vi "FCE_TS_Action_InitControls.vi"(8 "err in":errorcluster) -> (0 "err out":errorcluster)   [LabVIEW 2017]
uses:
  FCE_TS_General_Libs/WL_Libs_V14.25/WL_Alarm_V14.00.llb/WL_Alarm_TypeDefClusterStatus.ctl
  FCE_TS_GUI_V001.llb/FCE_TS_GUI_TDefEnumMessages.ctl
  FCE_TS_Auto_V001.llb/FCE_TS_Auto_TDefCluster_AutomaticSetpoints.ctl
  FCE_TS_Globals_V001.llb/Globals_Settings_FCE_TS.vi
  FCE_TS_Globals_V001.llb/FCE_TS_Globals_Status.vi
  FCE_TS_Globals_V001.llb/FCE_TS_Globals_Referenzen.vi
  FCE_TS_Alarm_V001.llb/FCE_TS_Alarm_Globals.vi
  FCE_TS_Auto_V001.llb/FCE_TS_Auto_Globals.vi
  FCE_TS_General_Libs/WL_Libs_V14.25/WL_Alarm_V14.00.llb/WL_Alarm_Globals.vi
  FCE_TS_Datalog_V002.llb/FCE_TS_Datalog_Globals.vi
  FCE_TS_General_Libs/WL_Libs_V14.25/WL_Profile_V14.00.llb/WL_Profile_Globals.vi
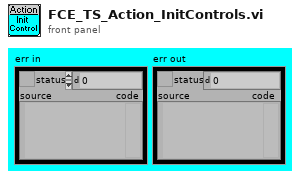
[diagram p1: front panel]
types:
  T1 = typedef "FCE_TS_Action_TDefEnumControl.ctl" = enum16{"Service", "Auto"}
  T2 = enum32{"Debug", "P&ID", "I/Os", "Regulator", "Datalog", "Automatic", "Charts", "CVM"}
  T3 = typedef "FCE_TS_GUI_TDefEnumMessages.ctl" = enum16{"Clear", "Add"}
  T4 = cluster{"Comment":string, "SamplingRate":u32, "Logging":bool, "FileName":string}
  T5 = typedef "FCE_TS_Auto_TDefCluster_AutomaticSetpoints.ctl" = cluster{"DC_Power":sgl, "AC_Power":sgl, "AC_Exists":bool, "Minute_Reserve":bool, "C_U_E_Soll":sgl, "Referenzpunkt_On":bool}
  T6 = typedef "WL_Alarm_TypeDefClusterStatus.ctl" = cluster{"NOTAUS":bool, "ABSCHALTEN":bool, "MELDUNG":bool}
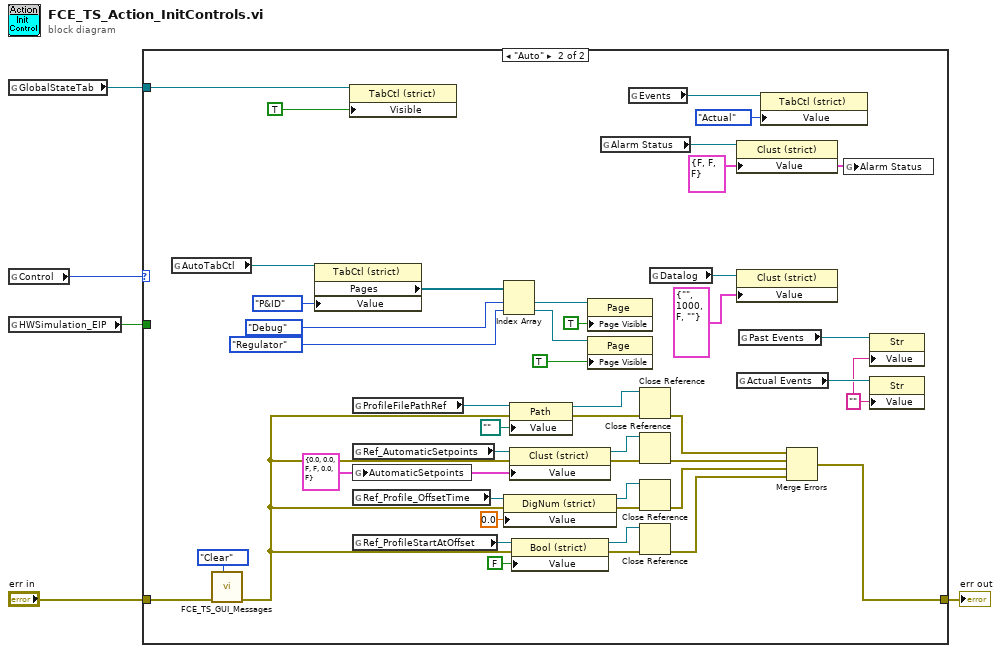
[diagram p0: block diagram]
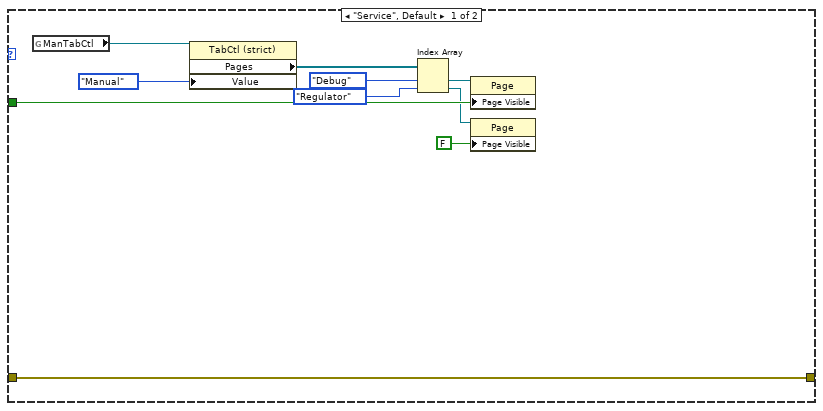
[diagram p2: hidden frame]
diagram:
  n1 = global read "FCE_TS_Globals_Referenzen.vi" "GlobalStateTab"() -> (w2:refnum<vi>)
  n2 = global read "FCE_TS_Globals_Status.vi" "Control"() -> (w3:T1)
  n3 = global read "Globals_Settings_FCE_TS.vi" "HWSimulation_EIP"() -> (w1:bool)
  n4 = case shown="\"Auto\"" w3 {
    tunnel: "err in" -> [w15 w59]
    tunnel: w1 -> [w11 _]
    tunnel: [w15 w35] -> w4
    tunnel: w2 -> [_ w46]
    frame "Service", Default {
      n5 = global read "FCE_TS_Globals_Referenzen.vi" "ManTabCtl"() -> (w14:refnum<vi>)
      n6 = property class="TabCtl (strict)"(reference=w14, "Value"=enum32{"Debug", "Manual", "Regulator"}."Manual") -> ("Pages"=w13:refnum<vi>[])  [unwired: 1 in, 2 out]
      n7 = Index Array(array=w13, index #1=enum32{"Debug", "Manual PCI", "Regulator"}."Debug" ("Value"), index #2=enum32{"Debug", "Manual PCI", "Regulator"}."Regulator" ("Value")) -> (element #1=w12:refnum<vi>, element #2=w10:refnum<vi>)
      n8 = property class="Page"(reference=w12, "Page Visible"=w11) -> ()  [unwired: 1 in, 2 out]
      n9 = property class="Page"(reference=w10, "Page Visible"=FALSE) -> ()  [unwired: 1 in, 2 out]
    }
    frame "Auto" {
      w39 = T5 {"DC_Power"=0.0, "AC_Power"=0.0, "AC_Exists"=FALSE, "Minute_Reserve"=FALSE, "C_U_E_Soll"=0.0, "Referenzpunkt_On"=FALSE} ("AutomaticSetpoints")
      w54 = T6 {"NOTAUS"=FALSE, "ABSCHALTEN"=FALSE, "MELDUNG"=FALSE} ("Alarm Status")
      w51 = "" ("Value")
      n10 = global read "FCE_TS_Globals_Referenzen.vi" "AutoTabCtl"() -> (w58:refnum<vi>)
      n11 = call "FCE_TS_GUI_Messages.vi"("Message"=FCE_TS_GUI_TDefEnumMessages."Clear", "err in"=w59) -> ("err out"=w21:errorcluster)  [unwired: 9 in]
      n12 = property class="TabCtl (strict)"(reference=w58, "Value"=T2."P&ID") -> ("Pages"=w57:refnum<vi>[])  [unwired: 1 in, 2 out]
      n13 = property class="TabCtl (strict)"(reference=w46, "Visible"=TRUE) -> ()  [unwired: 1 in, 2 out]
      n14 = global read "WL_Profile_Globals.vi" "ProfileFilePathRef"() -> (w33:refnum<vi>)
      n15 = global read "FCE_TS_Auto_Globals.vi" "Ref_AutomaticSetpoints"() -> (w40:refnum<vi>)
      n16 = global write "FCE_TS_Auto_Globals.vi" "AutomaticSetpoints"(w39) -> ()
      n17 = global read "FCE_TS_Auto_Globals.vi" "Ref_Profile_OffsetTime"() -> (w25:refnum<vi>)
      n18 = global read "FCE_TS_Auto_Globals.vi" "Ref_ProfileStartAtOffset"() -> (w23:refnum<vi>)
      n19 = Index Array(array=w57, index #1=T2."Debug" ("Value"), index #2=T2."Regulator" ("Value")) -> (element #1=w56:refnum<vi>, element #2=w43:refnum<vi>)
      n20 = property class="DigNum (strict)"(reference=w25, error in=w21, "Value"=sgl 0.0) -> (reference out=w29:refnum<vi>, error out=w28:errorcluster)
      n21 = property class="Path"(reference=w33, error in=w21, "Value"=path "") -> (reference out=w31:refnum<vi>, error out=w32:errorcluster)
      n22 = property class="Clust (strict)"(reference=w40, error in=w21, "Value"=w39) -> (reference out=w37:refnum<vi>, error out=w38:errorcluster)
      n23 = property class="Bool (strict)"(reference=w23, error in=w21, "Value"=FALSE) -> (reference out=w26:refnum<vi>, error out=w27:errorcluster)
      n24 = property class="Page"(reference=w56, "Page Visible"=TRUE) -> ()  [unwired: 1 in, 2 out]
      n25 = property class="Page"(reference=w43, "Page Visible"=TRUE) -> ()  [unwired: 1 in, 2 out]
      n26 = global read "WL_Alarm_Globals.vi" "Alarm Status"() -> (w55:refnum<vi>)
      n27 = global read "WL_Alarm_Globals.vi" "Events"() -> (w50:refnum<vi>)
      n28 = Close Reference(reference=w31, error in (no error)=w32) -> (error out=w30:errorcluster)
      n29 = Close Reference(reference=w37, error in (no error)=w38) -> (error out=w36:errorcluster)
      n30 = Close Reference(reference=w29, error in (no error)=w28) -> (error out=w20:errorcluster)
      n31 = Close Reference(reference=w26, error in (no error)=w27) -> (error out=w19:errorcluster)
      n32 = global read "FCE_TS_Datalog_Globals.vi" "Datalog"() -> (w48:refnum<vi>)
      n33 = property class="Clust (strict)"(reference=w55, "Value"=w54) -> ()  [unwired: 1 in, 2 out]
      n34 = property class="Clust (strict)"(reference=w48, "Value"=T4 {"Comment"="", "SamplingRate"=1000, "Logging"=FALSE, "FileName"=""}) -> ()  [unwired: 1 in, 2 out]
      n35 = global read "WL_Alarm_Globals.vi" "Actual Events"() -> (w52:refnum<vi>)
      n36 = global read "WL_Alarm_Globals.vi" "Past Events"() -> (w53:refnum<vi>)
      n37 = property class="TabCtl (strict)"(reference=w50, "Value"=enum32{"Actual", "Past"}."Actual") -> ()  [unwired: 1 in, 2 out]
      n38 = Merge Errors(w30, w36, w20, w19) -> (w35:errorcluster)
      n39 = global write "FCE_TS_Alarm_Globals.vi" "Alarm Status"(w54) -> ()
      n40 = property class="Str"(reference=w53, "Value"=w51) -> ()  [unwired: 1 in, 2 out]
      n41 = property class="Str"(reference=w52, "Value"=w51) -> ()  [unwired: 1 in, 2 out]
    }
  }
  "err out" <- w4
